vi "postScanHoldTime.vi"(8 "error in (no error)":errorcluster, 11 "GuassianNoiseWave in":refnum<class "GuassianNoiseWave.lvclass">) -> (0 "error out":errorcluster, 2 "PostscanHold?":bool=TRUE, 3 "GuassianNoiseWave out":refnum<class "GuassianNoiseWave.lvclass">)   [LabVIEW 2015, in "GuassianNoiseWave.lvclass"]
uses:
  GuassianNoiseWave.lvclass
  GuassianNoiseWave.lvclass/GuassianNoiseWave.ctl
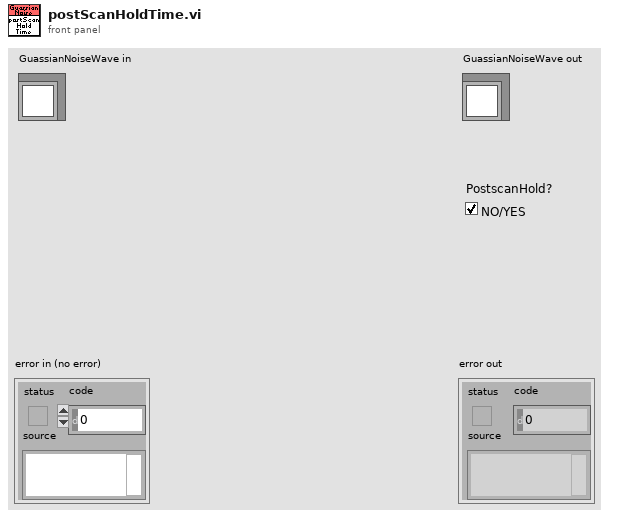
[diagram p1: front panel]
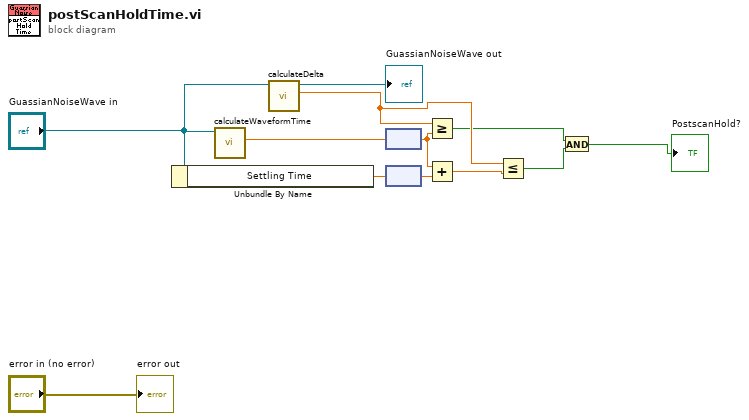
[diagram p0: block diagram]
diagram:
  n1 = Unbundle By Name("GuassianNoiseWave in") -> ("Settling Time"=w7:dbl[unit])
  n2 = call "calculateWaveformTime.vi"("GuassianNoiseWave in"="GuassianNoiseWave in") -> ("Waveform Time"=w9:dbl[unit])  [unwired: 8 in, 2 out]
  n3 = call "calculateDelta.vi"("GuassianNoiseWave in"="GuassianNoiseWave in") -> ("Delta Timestamp"=w5:dbl, "GuassianNoiseWave out"=→"GuassianNoiseWave out":refnum<class "GuassianNoiseWave.lvclass">)  [unwired: 8 in, 1 out]
  n4 = node(w9) -> (w8:dbl)
  n5 = node(w7) -> (w6:dbl)
  n6 = Greater Or Equal?(x=w5, y=w8) -> (x >= y?=w3:bool)
  n7 = Add(x=w8, y=w6) -> (x+y=w4:dbl)
  n8 = Less Or Equal?(x=w5, y=w4) -> (x <= y?=w2:bool)
  n9 = And(x=w3, y=w2) -> (x .and. y?=→"PostscanHold?":bool)
  "error out" <- "error in (no error)"
